vi "9093_第6回目課題_山口修平.vi"() -> ()   [LabVIEW 2020]
panel:
  out "運勢":string
  in  "OK Button":bool
  out "サイコロB":dbl
  out "サイコロA":dbl
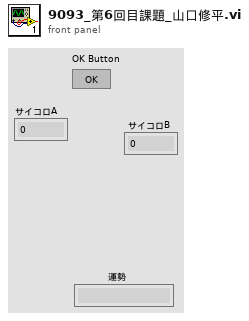
[diagram p1: front panel]
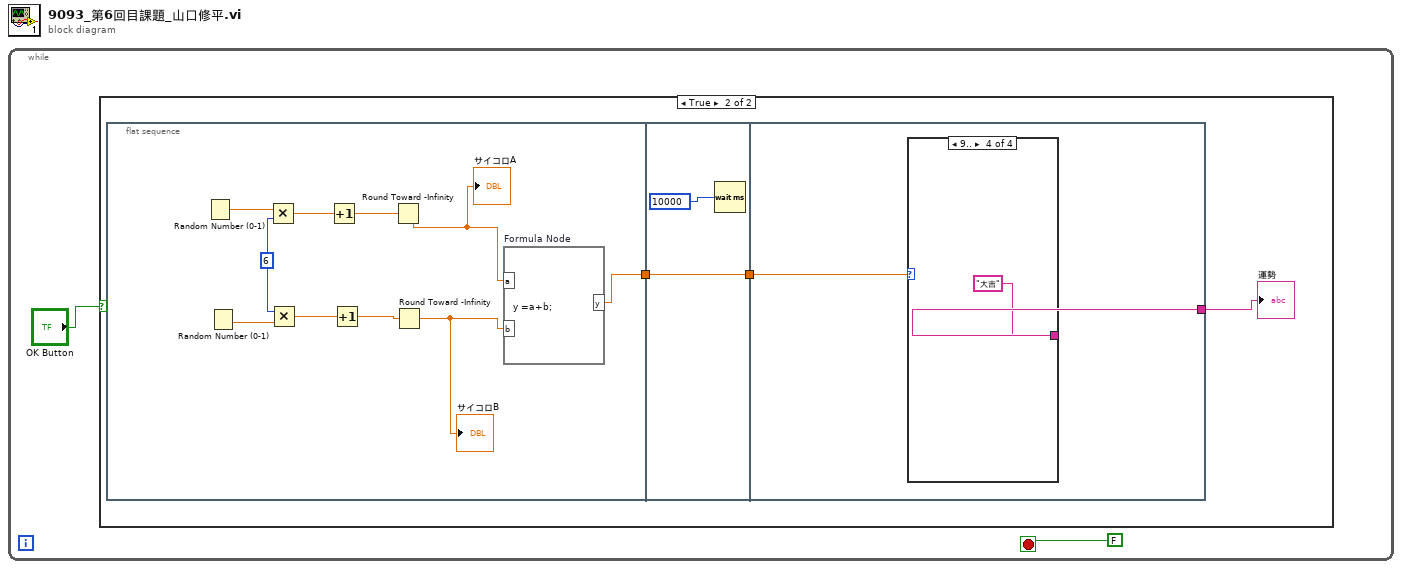
[diagram p0: block diagram]
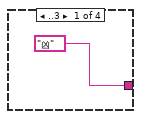
[diagram p3: hidden frame]
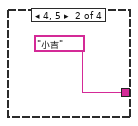
[diagram p4: hidden frame]
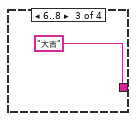
[diagram p5: hidden frame]
diagram:
  n1 = while {
    stop <- FALSE stop-if-true
    n2 = case shown="True" "OK Button" {
      frame False {
      }
      frame True {
        n3 = flat-sequence {
          tunnel: [w8] -> w4
          tunnel: [w17] -> w5
          tunnel: w4 -> [w17]
          tunnel: w5 -> [w19]
          tunnel: [w18] -> w3
          frame #0 {
            w14 = 6
            n4 = Random Number (0-1)() -> (number: 0 to 1=w15:dbl)
            n5 = Random Number (0-1)() -> (number: 0 to 1=w13:dbl)
            n6 = Multiply(x=w15, y=w14) -> (x*y=w12:dbl)
            n7 = Multiply(x=w14, y=w13) -> (x*y=w11:dbl)
            n8 = Increment(x=w12) -> (x+1=w9:dbl)
            n9 = Increment(x=w11) -> (x+1=w10:dbl)
            n10 = Round Toward -Infinity(1:w9) -> (0:w6:dbl)
            "サイコロA" <- w6
            n11 = Round Toward -Infinity(1:w10) -> (0:w7:dbl)
            "サイコロB" <- w7
            n12 = formula code="y =a+b;"("a"=w6, "b"=w7) -> ("y"=w8:dbl)
          }
          frame #1 {
            n13 = Wait (ms)(milliseconds to wait=10000) -> ()  [unwired: 1 out]
          }
          frame #2 {
            n14 = case shown="9.." w19 {
              tunnel: ["凶" ("文字列") "小吉" "大吉" "大吉"] -> w18
              frame ..3 {
              }
              frame 4, 5 {
              }
              frame 6..8 {
              }
              frame 9.. {
              }
            }
          }
        }
        "運勢" <- w3
      }
    }
  }
